vi "Initialize Tree with Plugins.vi"(8 "error in (no error)":errorcluster, 11 "Application Data in":T1) -> (0 "error out":errorcluster, 3 "Application Data out":T1)   [LabVIEW 2017, in "DSF Configuration Utility.lvlib"]
uses:
  DSF Configuration Utility.lvlib
  Application Data.ctl
  VeriStand/Data Sharing Custom Device/Source/DSF Core.lvlibp/DSF Configuration API/Configuration Session.lvclass
  View Mode.ctl
  Item Tree/Tree Item.ctl
  Item Tree/ID to Tree Items/Plugin ID to Tree Items.vi
  Item Tree/Create New Tree Item.vi
  VeriStand/Data Sharing Custom Device/Source/DSF Core.lvlibp/DSF Configuration API/Public/Read Item.vi
  VeriStand/Data Sharing Custom Device/Source/DSF Core.lvlibp/DSF Configuration API/Public/Read Item/Read Settings.vi
  VeriStand/Data Sharing Custom Device/Source/DSF Core.lvlibp/DSF Configuration API/Public/Read Item/Read Plugin.vi
  VeriStand/Data Sharing Custom Device/Source/DSF Core.lvlibp/DSF Configuration API/Public/Read All Item IDs/Read All Plugin IDs.vi
panel:
  # "App\nData"
  # "App\nData"
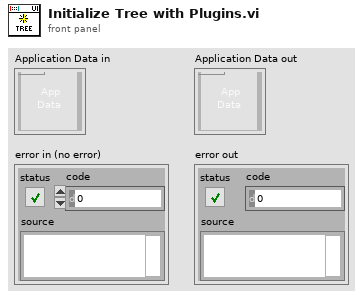
[diagram p1: front panel]
types:
  T1 = typedef "DSF Configuration Utility.lvlib/Application Data.ctl" = cluster{"Item Tree Control":refnum<vi>, "Value Tree Control":refnum<vi>, "DSF Refnum":refnum<class "Configuration Session.lvclass">, "Top-Level VI":refnum<vi>, "View State":T2, "menu reference":refnum<k9>}
  T2 = typedef "DSF Configuration Utility.lvlib/View Mode.ctl" = enum16{"Tree", "List"}
  T3 = typedef "DSF Configuration Utility.lvlib/Tree Item.ctl" = cluster{"Left Cell String":string, "Child Text":string[], "Child Tag":string, "Glyph Index":i32}
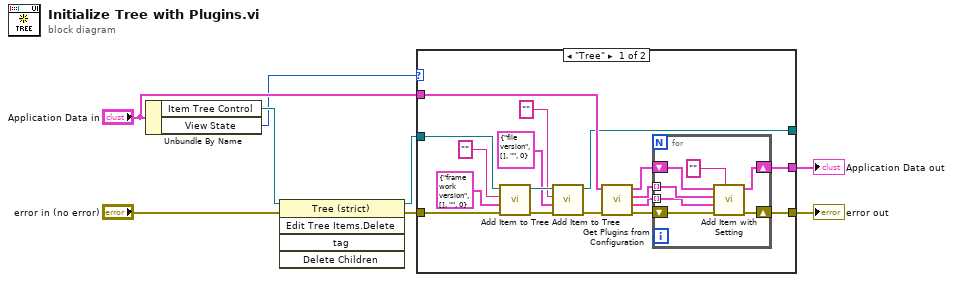
[diagram p0: block diagram]
diagram:
  n1 = Unbundle By Name("Application Data in") -> ("Item Tree Control"=w2:refnum<vi>, "View State"=w1:T2)
  n2 = invoke class="Tree (strict)" method="Edit Tree Items.Delete"(reference=w2, error in="error in (no error)") -> (reference out=w5:refnum<vi>, error out=w6:errorcluster)  [unwired: 3 in, 3 out]
  n3 = case shown="\"Tree\"" w1 {
    tunnel: "Application Data in" -> [w25 w35]
    tunnel: w6 -> [w24 w34]
    tunnel: w5 -> [w15 w33]
    tunnel: [w9 w33] -> _
    tunnel: [w20 w34] -> w4
    tunnel: [w22 w35] -> w3
    frame "Tree" {
      n4 = call "Add Item to Tree.vi"("error in (no error)"=w24, "Item"=T3 {"Left Cell String"="framework version", "Child Text"=[], "Child Tag"="", "Glyph Index"=0}, "parent tag"="", "TreeControl in"=w15) -> ("error out"=w16:errorcluster, "TreeControl out"=w14:refnum<vi>)  [unwired: 5 in, 1 out]
      n5 = call "Add Item to Tree.vi"("error in (no error)"=w16, "Item"=T3 {"Left Cell String"="file version", "Child Text"=[], "Child Tag"="", "Glyph Index"=0}, "parent tag"="", "TreeControl in"=w14) -> ("error out"=w17:errorcluster, "TreeControl out"=w9:refnum<vi>)  [unwired: 5 in, 1 out]
      n6 = call "Get Plugins from Configuration.vi"("error in (no error)"=w17, "Application Data In"=w25) -> ("error out"=w21:errorcluster, "Settings"=w18:T3[], "Items"=w19:T3[], "Application Data out"=w23:T1)  [unwired: 6 in]
      n7 = for {
        shift-right: [w31] -> w22
        shift-left: w23 -> [w32]
        shift-right: [w29] -> w20
        shift-left: w21 -> [w30]
        tunnel: w19 -> [w27] mode=indexing
        tunnel: w18 -> [w26] mode=indexing
        n8 = call "Add Item with Setting.vi"("Tag"="", "error in (no error)"=w30, "Setting"=w26, "Item"=w27, "Application Data in"=w32) -> ("error out"=w29:errorcluster, "Application Data out"=w31:T1)  [unwired: 4 in, 1 out]
      }
    }
    frame "List" {
    }
  }
  "error out" <- w4
  "Application Data out" <- w3
